vi "Image Comparison Score.vi"(10 "Image 2":path caption="Image 2 (Altered Image)", 11 "Image 1":path caption="Image 1 (Original Image)") -> (3 "Composite Score":dbl)   [LabVIEW 2015]
uses:
  HSV Distance Comparison/HSV Distance Comparison.lvclass
  Histogram Comparison/Histogram Comparison.lvclass
  Histogram Grid Comparison/Histogram Grid Comparison.lvclass
  RGB Distance Comparison/RGB Distance Comparison.lvclass
  Difference Comparision/Difference Comparision.lvclass
  Perceptual Hash Comparison/Perceptual Hash Comparison.lvclass
panel:
  out "RGB Distance":dbl
  out "Histogram Grid":dbl
  out "pHash Cross Correlation":dbl
  out "File Size Difference":dbl
  out "Differencing":dbl
  out "Histogram":dbl
  out "HSV Distance":dbl
  # "Closer to 0 the better"
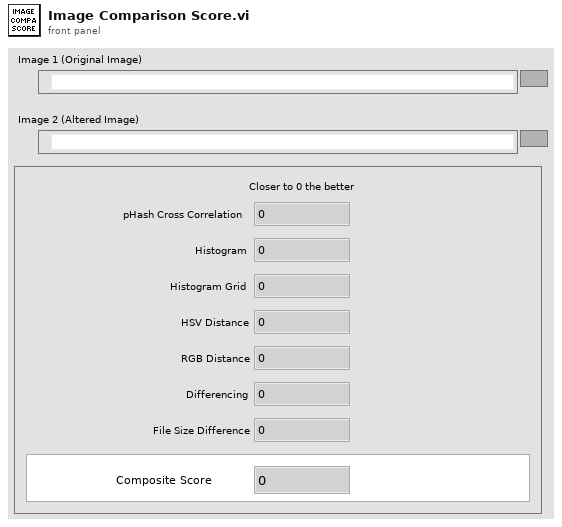
[diagram p1: front panel]
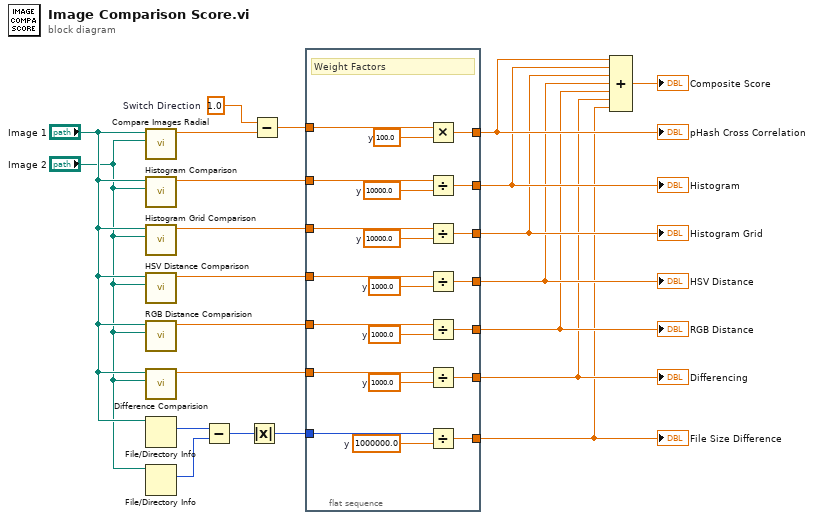
[diagram p0: block diagram]
diagram:
  w19 = 1.0  # Switch Direction
  n1 = call "Compare Images Radial.vi"("Image 2"="Image 2", "Image 1"="Image 1") -> ("Perceptual Cross Correlation"=w1:dbl)  [unwired: 9 in]
  n2 = call "Histogram Comparison.vi"("Image 2"="Image 2", "Image 1"="Image 1") -> ("Histogram Comparison Score"=w16:dbl)  [unwired: 7 in, 2 out]
  n3 = call "Histogram Grid Comparison.vi"("Image 2"="Image 2", "Image 1"="Image 1") -> ("Histogram Grid Comparison Score"=w15:dbl)  [unwired: 7 in, 2 out]
  n4 = call "HSV Distance Comparison.vi"("Image 2"="Image 2", "Image 1"="Image 1") -> ("HSV Distance"=w14:dbl)  [unwired: 9 in]
  n5 = call "RGB Distance Comparision.vi"("Image 2"="Image 2", "Image 1"="Image 1") -> ("RGB Distance"=w13:dbl)  [unwired: 9 in]
  n6 = call "Difference Comparision.vi"("Image 2"="Image 2", "Image 1"="Image 1") -> ("Difference"=w12:dbl)  [unwired: 9 in]
  n7 = File/Directory Info(path="Image 1") -> (size=w22:i64)  [unwired: 1 in, 6 out]
  n8 = File/Directory Info(path="Image 2") -> (size=w21:i64)  [unwired: 1 in, 6 out]
  n9 = Subtract(x=w22, y=w21) -> (x-y=w20:i64)
  n10 = Absolute Value(x=w20) -> (abs(x)=w11:i64)
  n11 = Subtract(x=w19, y=w1) -> (x-y=w18:dbl)
  n12 = flat-sequence {
    tunnel: w18 -> [w43]
    tunnel: w16 -> [w41]
    tunnel: w15 -> [w38]
    tunnel: w14 -> [w36]
    tunnel: w13 -> [w34]
    tunnel: w12 -> [w32]
    tunnel: w11 -> [w30]
    tunnel: [w29] -> w10
    tunnel: [w28] -> w9
    tunnel: [w27] -> w8
    tunnel: [w26] -> w7
    tunnel: [w25] -> w6
    tunnel: [w24] -> w5
    tunnel: [w23] -> w4
    frame #0 {
      w31 = 1000000.0  # y
      w33 = 1000.0  # y
      w35 = 1000.0  # y
      w37 = 1000.0  # y
      w39 = 10000.0  # y
      w40 = 10000.0  # y
      w42 = 100.0  # y
      # "Weight Factors"
      n13 = Multiply(x=w43, y=w42) -> (x*y=w29:dbl)
      n14 = Divide(x=w41, y=w40) -> (x/y=w28:dbl)
      n15 = Divide(x=w38, y=w39) -> (x/y=w27:dbl)
      n16 = Divide(x=w36, y=w37) -> (x/y=w26:dbl)
      n17 = Divide(x=w34, y=w35) -> (x/y=w25:dbl)
      n18 = Divide(x=w32, y=w33) -> (x/y=w24:dbl)
      n19 = Divide(x=w30, y=w31) -> (x/y=w23:dbl)
    }
  }
  n20 = Compound Arithmetic op=ADD(w10, w9, w8, w7, w6, w5, w4) -> (→"Composite Score":dbl)
  "HSV Distance" <- w7
  "Histogram" <- w9
  "Differencing" <- w5
  "File Size Difference" <- w4
  "pHash Cross Correlation" <- w10
  "Histogram Grid" <- w8
  "RGB Distance" <- w6
